vi "InitBurstTriggers.vi"(9 "metric ids":string[](array[string]), 11 "device configuration":T1) -> (1 "valid config":bool, 2 "device":T12)   [LabVIEW 2017, in "BurstMode.lvlib"]
uses:
  <vilib>/addons/InsightCM/Devices/Shared/Cms/CmsBurstMode/BurstMode.lvlib
  <vilib>/addons/InsightCM/Devices/Shared/Cms/CmsBurstMode/controls/device.ctl
  <vilib>/addons/InsightCM/MessageBus/Base/controls/KeyValuePair.ctl
  <vilib>/addons/InsightCM/Devices/Shared/Common/Trigger/controls/TriggerCondition.ctl
  <vilib>/addons/InsightCM/MessageBus/Base/controls/Condition.ctl
  <vilib>/addons/InsightCM/MessageBus/Base/controls/R2_Device.ctl
  <vilib>/addons/InsightCM/MessageBus/Base/controls/DeviceState.ctl
  <vilib>/addons/InsightCM/MessageBus/Base/controls/R2_DataGroup.ctl
  <vilib>/addons/InsightCM/MessageBus/Base/controls/OperatingState.ctl
  <vilib>/addons/InsightCM/MessageBus/Base/controls/Trigger.ctl
  <vilib>/addons/InsightCM/MessageBus/Base/controls/BurstModeTrigger.ctl
  <vilib>/addons/InsightCM/MessageBus/Base/controls/DeviceSensorGroup.ctl
  <vilib>/addons/InsightCM/MessageBus/Base/controls/WirelessEndpoint.ctl
  <vilib>/addons/InsightCM/MessageBus/Base/controls/WirelessChannel.ctl
  <vilib>/addons/InsightCM/Devices/Shared/Common/Trigger/Trigger.lvlib
  <vilib>/addons/InsightCM/Devices/Shared/Common/OpState/OpState.lvlib
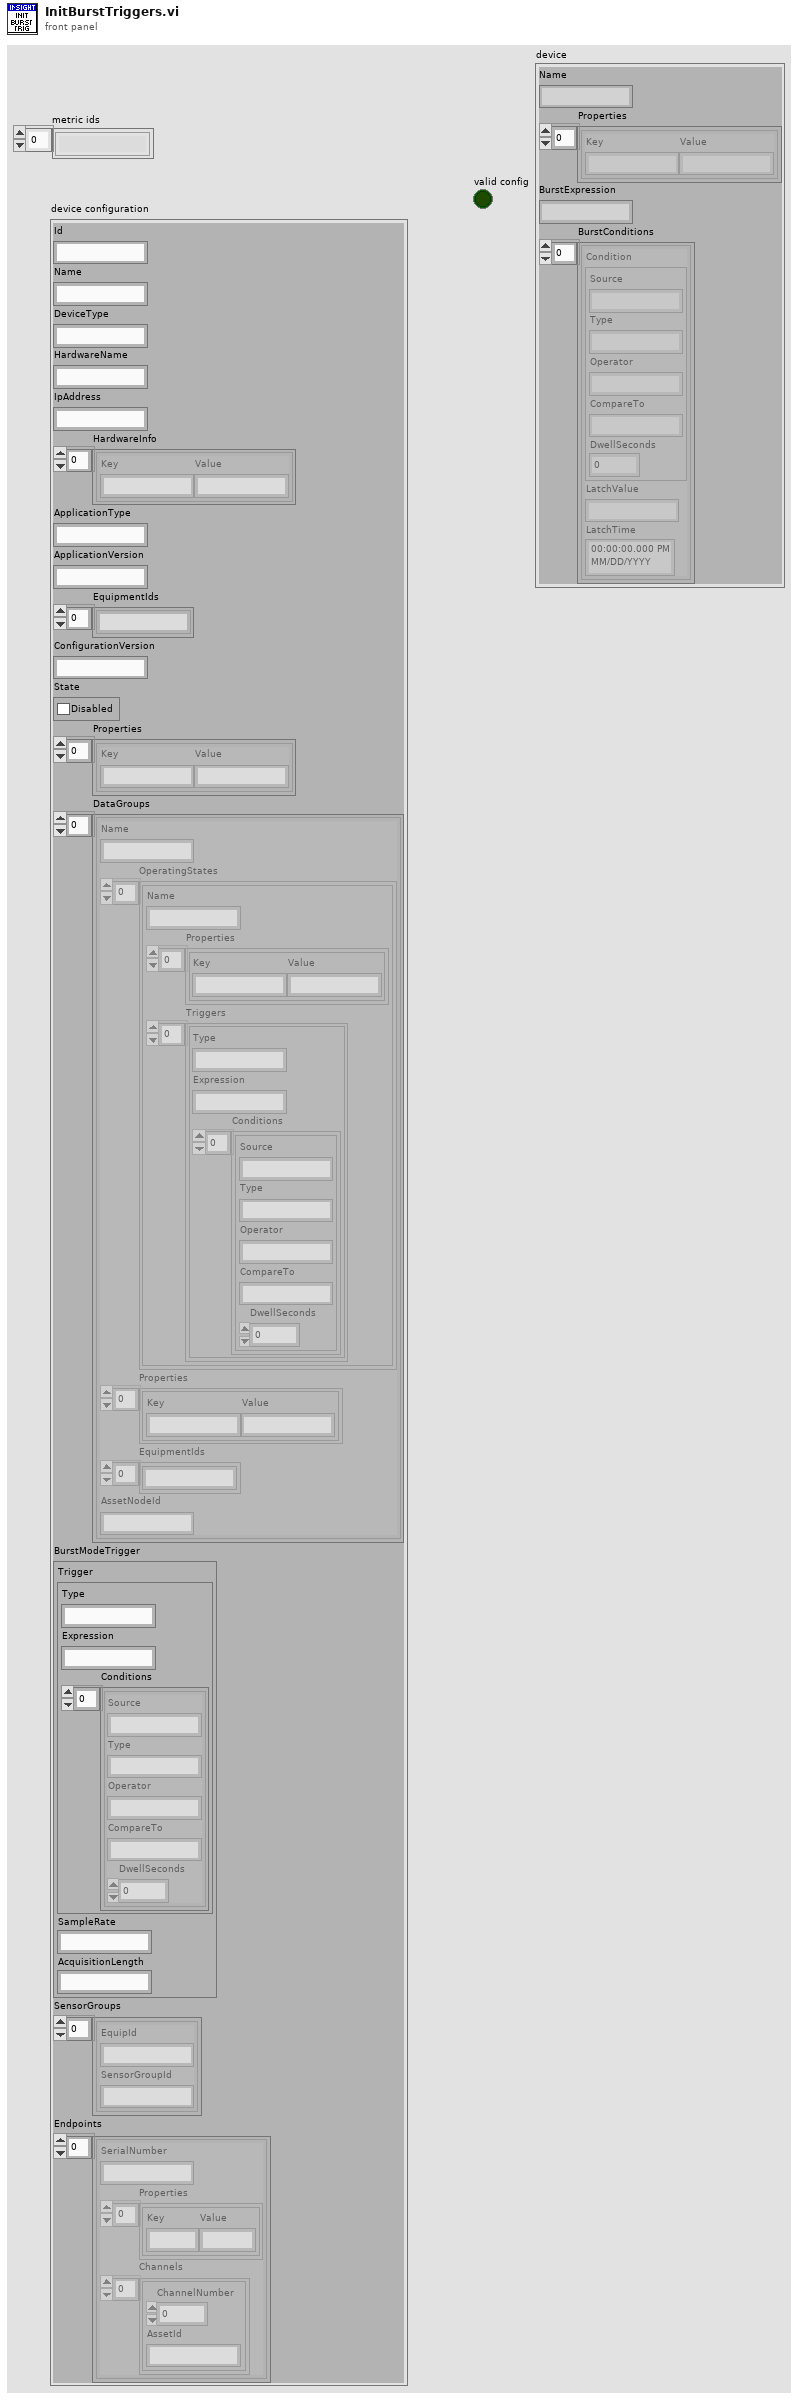
[diagram p1: front panel]
types:
  T1 = typedef "R2_Device.ctl" = cluster{"Id":string, "Name":string, "DeviceType":string, "HardwareName":string, "IpAddress":string, "HardwareInfo":T2[], "ApplicationType":string, "ApplicationVersion":string, "EquipmentIds":string[], "ConfigurationVersion":string, "State":T3, "Properties":T2[], "DataGroups":T4[], "BurstModeTrigger":T8, "SensorGroups":T9[], "Endpoints":T10[]}
  T2 = typedef "KeyValuePair.ctl" = cluster{"Key":string, "Value":string}
  T3 = typedef "DeviceState.ctl" = cluster{"Disabled":bool}
  T4 = typedef "R2_DataGroup.ctl" = cluster{"Name":string, "OperatingStates":T5[], "Properties":T2[], "EquipmentIds":string[], "AssetNodeId":string}
  T5 = typedef "OperatingState.ctl" = cluster{"Name":string, "Properties":T2[], "Triggers":T6[]}
  T6 = typedef "Trigger.ctl" = cluster{"Type":string, "Expression":string, "Conditions":T7[]}
  T7 = typedef "Condition.ctl" = cluster{"Source":string, "Type":string, "Operator":string, "CompareTo":string, "DwellSeconds":dbl}
  T8 = typedef "BurstModeTrigger.ctl" = cluster{"Trigger":T6, "SampleRate":string, "AcquisitionLength":string}
  T9 = typedef "DeviceSensorGroup.ctl" = cluster{"EquipId":string, "SensorGroupId":string}
  T10 = typedef "WirelessEndpoint.ctl" = cluster{"SerialNumber":string, "Properties":T2[], "Channels":T11[]}
  T11 = typedef "WirelessChannel.ctl" = cluster{"ChannelNumber":i32, "AssetId":string}
  T12 = typedef "BurstMode.lvlib/device.ctl" = cluster{"Name":string, "Properties":T2[], "BurstExpression":string, "BurstConditions":T13[]}
  T13 = typedef "Trigger.lvlib/TriggerCondition.ctl" = cluster{"Condition":T7, "LatchValue":string, "LatchTime":timestamp}
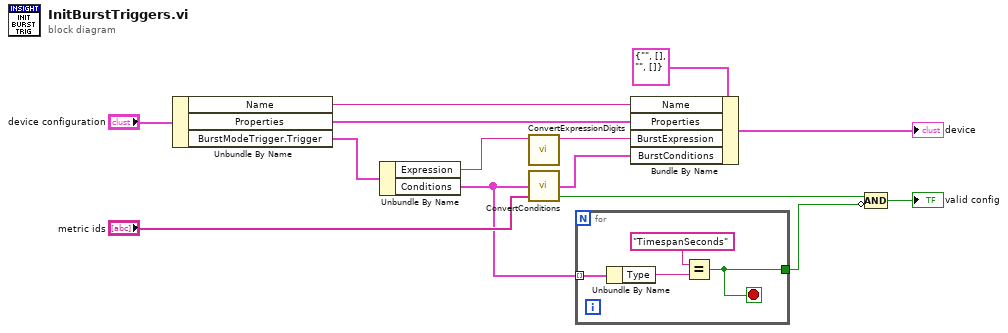
[diagram p0: block diagram]
diagram:
  n1 = Unbundle By Name("device configuration") -> ("Name"=w14:string, "Properties"=w13:T2[], "BurstModeTrigger.Trigger"=w1:T6)
  n2 = Unbundle By Name(w1) -> ("Expression"=w11:string, "Conditions"=w4:T7[])
  n3 = call <vilib>:"ConvertExpressionDigits.vi"("input"=w11) -> ("output"=w10:string)  [unwired: 10 in]
  n4 = call <vilib>:"ConvertConditions.vi"("metric ids"="metric ids", "conditions"=w4) -> ("valid config"=w6:bool, "trigger conditions"=w12:T13[])  [unwired: 2 in]
  n5 = for {
    tunnel: w4 -> [w18] mode=indexing
    tunnel: [w15] -> w9
    stop <- w15 stop-if-true
    n6 = Unbundle By Name(w18) -> ("Type"=w17:string)
    n7 = Equal?(x="TimespanSeconds", y=w17) -> (x = y?=w15:bool)
  }
  n8 = Bundle By Name(cluster=T12 {"Name"="", "Properties"=[], "BurstExpression"="", "BurstConditions"=[]} ("Device Burst Mode"), "Name"=w14, "Properties"=w13, "BurstExpression"=w10, "BurstConditions"=w12) -> (→"device":T12)
  n9 = Compound Arithmetic op=AND(w6, invert w9) -> (→"valid config":bool)
